vi "test_MonoGrating.vi"(8 "error in":errorcluster, 11 "Monochromator in":refnum<class "Monochromator.lvclass">) -> (0 "error out":errorcluster, 2 "iterations":i32, 3 "Monochromator out":refnum<class "Monochromator.lvclass">)   [LabVIEW 2020, in "horiba.test.lvlib"]
uses:
  horiba.test.lvlib
  Classes/Mono/Monochromator.lvclass
  <vilib>/addons/_JKI Toolkits/Caraya/classes/Assert/Assert Equal Value_Variant.vi
panel:
  # "Connector Pane"
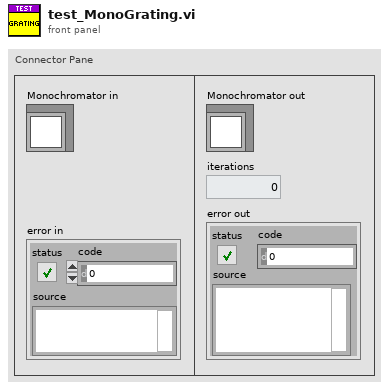
[diagram p1: front panel]
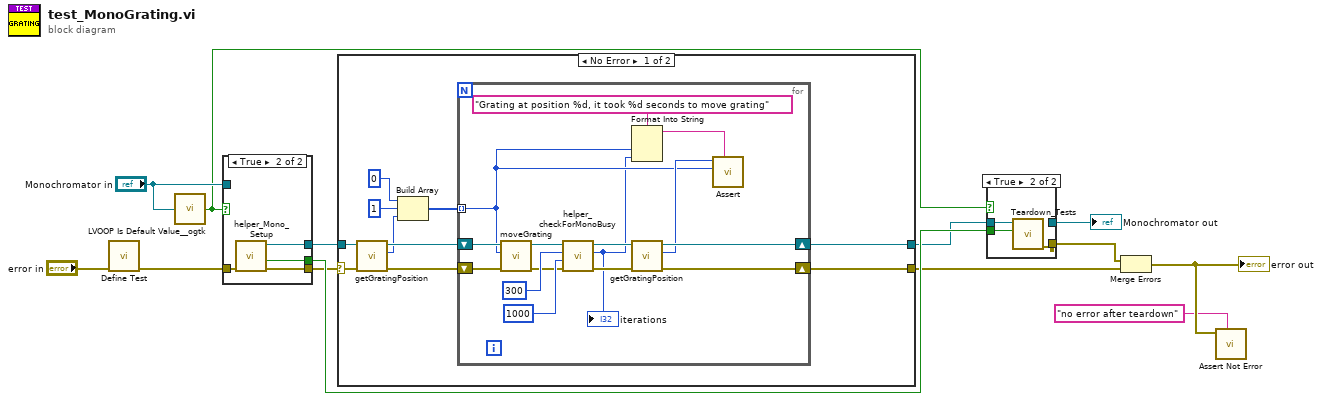
[diagram p0: block diagram]
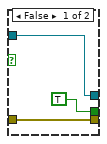
[diagram p2: hidden frame]
diagram:
  n1 = call <vilib>:"Define Test.vi"("error in (no error)"="error in") -> ("error out"=w7:errorcluster)  [unwired: 9 in, 1 out]
  n2 = call <userlib>:"LVOOP Is Default Value__ogtk.vi"("Object"="Monochromator in") -> ("Is Default Value?"=w8:bool)
  n3 = case shown="True" w8 {
    tunnel: w7 -> [w15 w20]
    tunnel: [w15 w19] -> w2
    tunnel: [w16 w18] -> w5
    tunnel: [TRUE ("Module Was Already Running?") w17] -> w10
    tunnel: "Monochromator in" -> [w16 _]
    frame False {
    }
    frame True {
      n4 = call "helper_Mono_Setup.vi"("error in"=w20) -> ("error out"=w19:errorcluster, "Module Was Already Running?"=w17:bool, "Monochromator out"=w18:refnum<class "Monochromator.lvclass">)  [unwired: 7 in, 1 out]
    }
  }
  n5 = case shown="No Error" w2 {
    selector: w2 -> [w29 w47]
    tunnel: [w25 w46] -> w4
    tunnel: w5 -> [w30 w46]
    tunnel: [w26 w47] -> w1
    frame No Error {
      n6 = call "getGratingPosition.vi"("error in (no error)"=w29, "Monochromator in"=w30) -> ("error out"=w28:errorcluster, "Position"=w22:i32, "Monochromator out"=w27:refnum<class "Monochromator.lvclass">)  [unwired: 7 in]
      n7 = Build Array(0 ("position"), 1 ("element"), w22) -> (w23:i32[])
      n8 = for {
        tunnel: w23 -> [w33] mode=indexing
        shift-right: [w38] -> w26
        shift-left: w28 -> [w45]
        shift-right: [w36] -> w25
        shift-left: w27 -> [w40]
        n9 = call "moveGrating.vi"("error in (no error)"=w45, "position"=w33, "Monochromator in"=w40) -> ("error out"=w41:errorcluster, "Monochromator out"=w39:refnum<class "Monochromator.lvclass">)  [unwired: 5 in, 2 out]
        n10 = call "helper_checkForMonoBusy.vi"("error in (no error)"=w41, "milliseconds to wait"=u32 1000, "Numeric"=300, "Monochromator in"=w39) -> ("error out"=w42:errorcluster, "iterations"=w32:i32, "Monochromator out"=w37:refnum<class "Monochromator.lvclass">)  [unwired: 5 in]
        "iterations" <- w32
        n11 = Format Into String(format string="Grating at position %d, it took %d seconds to move grating", w33, w32) -> (resulting string=w31:string)  [unwired: 2 in, 1 out]
        n12 = call "getGratingPosition.vi"("error in (no error)"=w42, "Monochromator in"=w37) -> ("error out"=w38:errorcluster, "Position"=w35:i32, "Monochromator out"=w36:refnum<class "Monochromator.lvclass">)  [unwired: 7 in]
        n13 = call-poly <vilib>:"Assert.vi"("Label"=w31, "Y"=w33, "X"=w35) -> ()  [unwired: 7 in, 2 out]
      }
    }
    frame Error {
    }
  }
  n14 = case shown="True" w8 {
    tunnel: w4 -> [w48 w51]
    tunnel: [_ w50] -> w6
    tunnel: w10 -> [_ w49]
    tunnel: [w48 _] -> w3
    frame False {
    }
    frame True {
      n15 = call "Teardown_Tests.vi"("Module Was Already Running?"=w49, "horiba.lvlib:GenericDevice"=w51) -> ("error out"=w50:errorcluster)  [unwired: 8 in, 1 out]
    }
  }
  "Monochromator out" <- w3
  n16 = Merge Errors(w6, w1) -> (w12:errorcluster)
  "error out" <- w12
  n17 = call <vilib>:"Assert Not Error.vi"("Label"="no error after teardown", "Not Error?"=w12) -> ()  [unwired: 8 in, 2 out]
